vi "Mode Page.vi"(8 "Error in":errorcluster, 11 "INL DNL Test in":refnum<class "INL DNL Test.lvclass">) -> (0 "Error out":errorcluster, 3 "INL DNL Test out":refnum<class "INL DNL Test.lvclass">)   [LabVIEW 2020, in "INL DNL Test.lvclass"]
uses:
  INL DNL Test.lvclass
  D:/SDLC/Class/INL DNL Test/Test/Parent/Test.lvclass
  Typedef/User event controls.ctl
  Device/Parent/Device.lvclass
  DNL INL Test.lvlib
panel:
  out "number (0 to 1)":dbl
  in  "Error Rate":dbl
  in  "Voltage":dbl
  in  "Resolution":dbl
  in  "Digital to Analog converter":bool
  in  "Analog to digital converter":bool
  # "Choose the mode"
  # "Enter parameters"
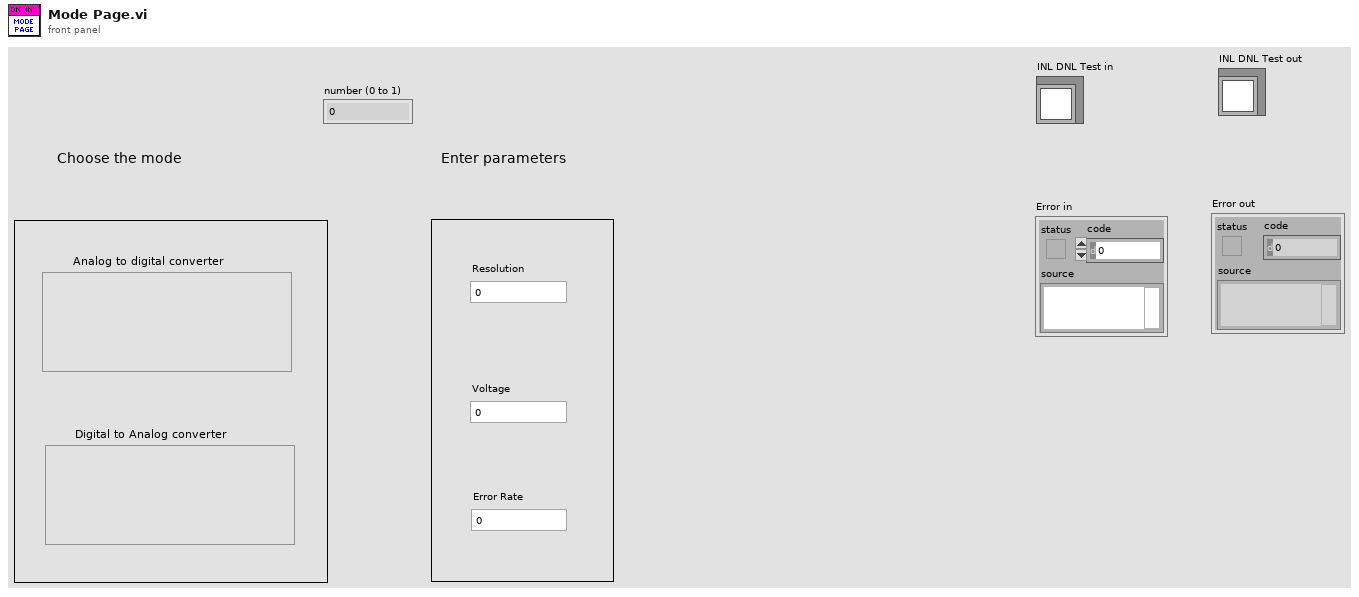
[diagram p1: front panel]
types:
  T1 = typedef "DNL INL Test.lvlib/User event controls.ctl" = enum16{"Create", "Generate", "Get Ref", "Destroy"}
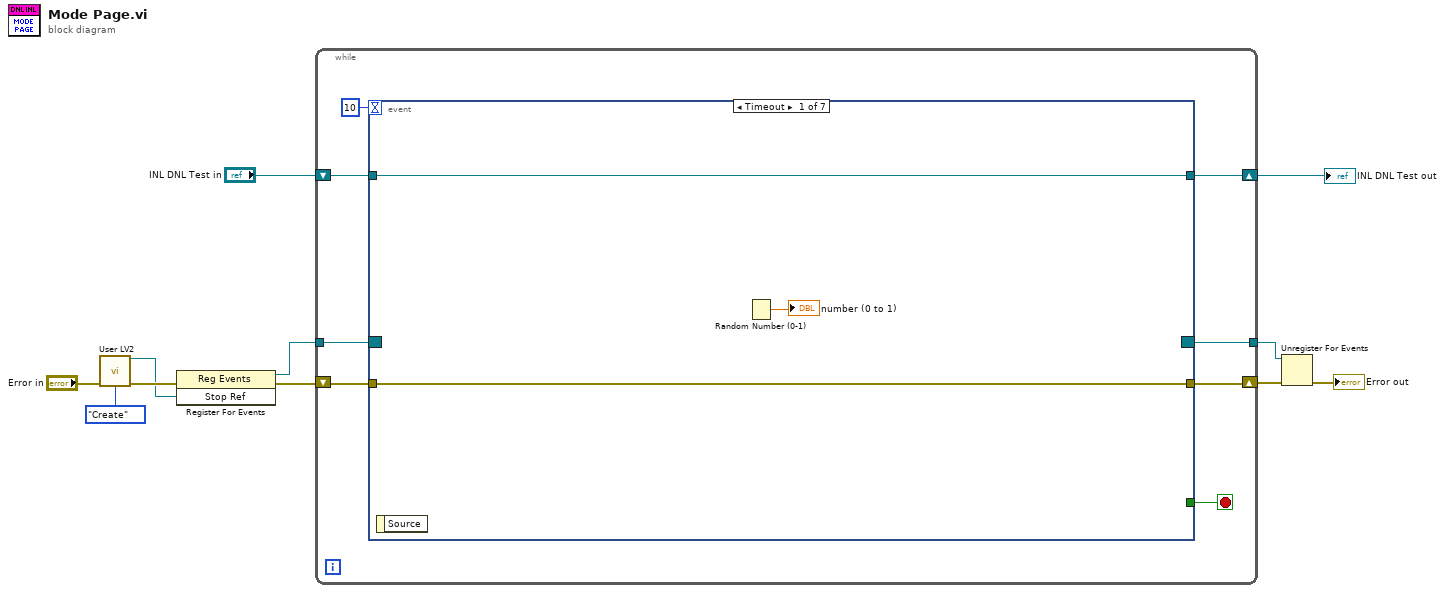
[diagram p0: block diagram]
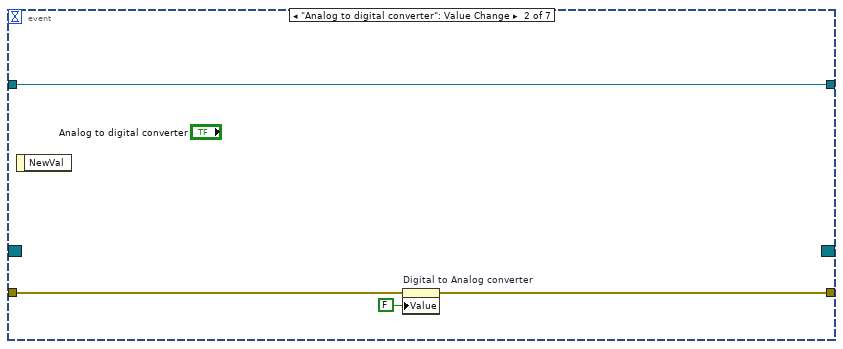
[diagram p2: hidden frame]
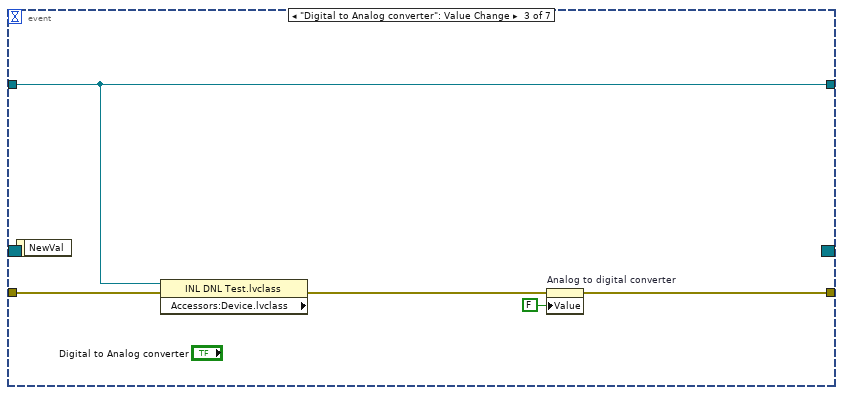
[diagram p3: hidden frame]
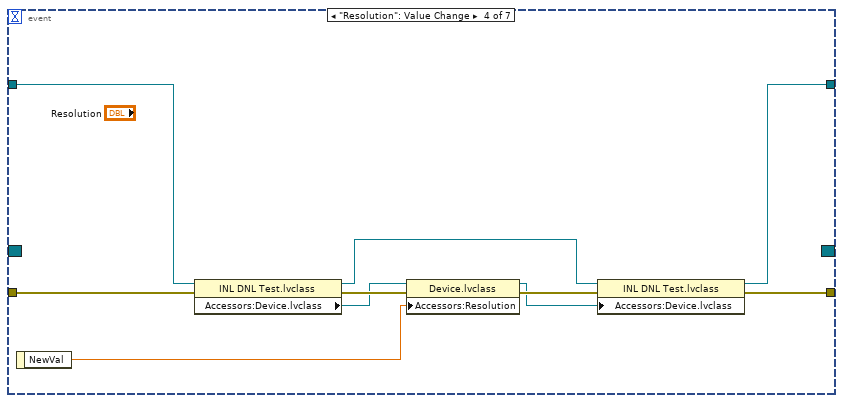
[diagram p4: hidden frame]
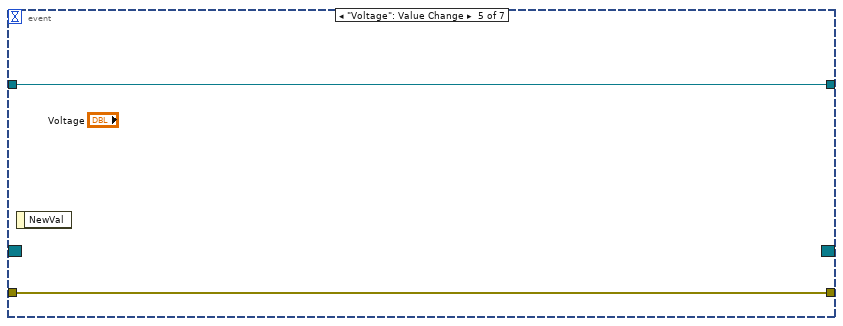
[diagram p5: hidden frame]
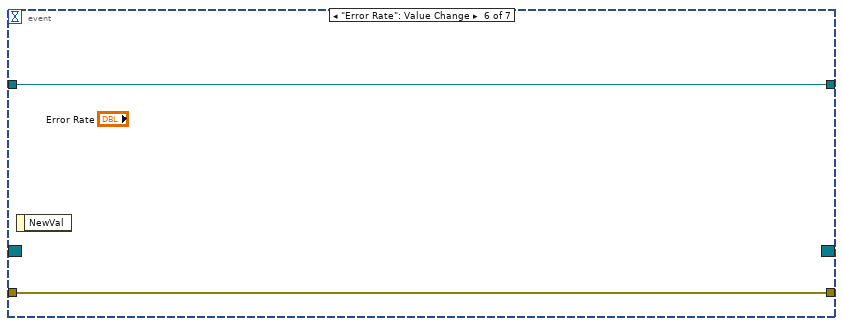
[diagram p6: hidden frame]
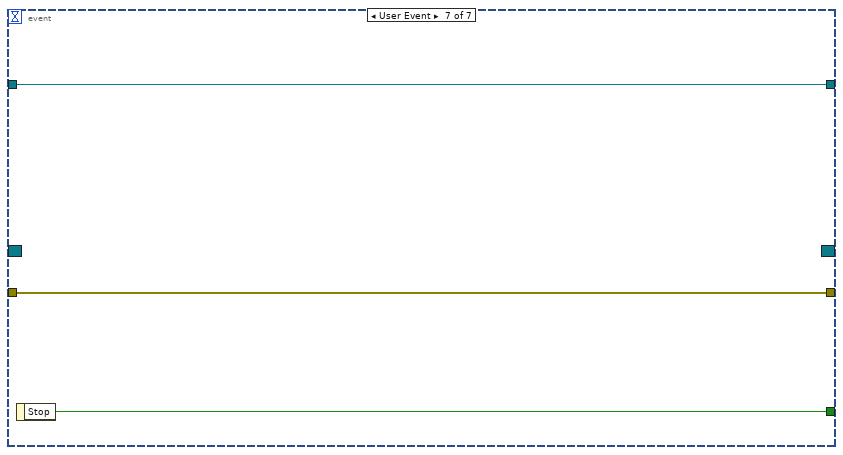
[diagram p7: hidden frame]
diagram:
  n1 = call "User LV2.vi"("Error In"="Error in", "User event controls"=User_event_controls."Create") -> ("Stop Ref"=w8:refnum<user-event>, "Error Out"=w9:errorcluster)  [unwired: 12 in]
  n2 = register-events(error in=w9, w8) -> (reference out=w7:refnum<event-registration>, error out=w6:errorcluster)  [unwired: 1 in]
  n3 = while {
    tunnel: w7 -> [w18]
    shift-right: [w15] -> w4
    shift-left: "INL DNL Test in" -> [w16]
    shift-right: [w13] -> w3
    shift-left: w6 -> [w17]
    tunnel: [w12] -> w1
    stop <- w14 stop-if-true
    n4 = event shown="[0] Timeout" {
      selector: w18 -> [_ _ _ _ _ _ _]
      dyn-events: [_ _ _ _ _ _ _] -> w12
      timeout: 10 -> [_ _ _ _ _ _ _]
      tunnel: w17 -> [w21 w25 w31 w41 w42 w44 w46]
      tunnel: w16 -> [w22 w26 w29 w39 w43 w45 w48]
      tunnel: [w22 w26 w29 w32 w43 w45 w48] -> w15
      tunnel: [_ _ _ _ _ _ w47] -> w14
      tunnel: [w21 w24 w28 w35 w42 w44 w46] -> w13
      event Timeout {
        n5 = event-data() -> ()  [unwired: 1 in, 1 out]
        n6 = Random Number (0-1)() -> (number: 0 to 1=→"number (0 to 1)":dbl)
      }
      event "Analog to digital converter": Value Change {
        n7 = event-data() -> ()  [unwired: 1 in, 1 out]
        n8 = property on="Digital to Analog converter" class="Bool (strict)"(error in=w25, "Value"=FALSE ("Digital to Analog converter")) -> (error out=w24:errorcluster)  [unwired: 1 in, 1 out]
      }
      event "Digital to Analog converter": Value Change {
        n9 = event-data() -> ()  [unwired: 1 in, 1 out]
        n10 = property class="INL DNL Test.lvclass" props=["Accessors:Device.lvclass"](reference=w29, error in=w31) -> (error out=w30:errorcluster)  [unwired: 2 out]
        n11 = property on="Analog to digital converter" class="Bool (strict)"(error in=w30, "Value"=FALSE ("Analog to digital converter")) -> (error out=w28:errorcluster)  [unwired: 1 in, 1 out]
      }
      event "Resolution": Value Change {
        n12 = event-data() -> ("NewVal"=w36:dbl)  [unwired: 1 in]
        n13 = property class="INL DNL Test.lvclass"(reference=w39, error in=w41) -> (reference out=w34:refnum<class "INL DNL Test.lvclass">, error out=w40:errorcluster, "Accessors:Device.lvclass"=w37:refnum<class "Device.lvclass">)
        n14 = property class="Device.lvclass"(reference=w37, error in=w40, "Accessors:Resolution"=w36) -> (reference out=w33:refnum<class "Device.lvclass">, error out=w38:errorcluster)
        n15 = property class="INL DNL Test.lvclass"(reference=w34, error in=w38, "Accessors:Device.lvclass"=w33) -> (reference out=w32:refnum<class "INL DNL Test.lvclass">, error out=w35:errorcluster)
      }
      event "Voltage": Value Change {
        n16 = event-data() -> ()  [unwired: 1 in, 1 out]
      }
      event "Error Rate": Value Change {
        n17 = event-data() -> ()  [unwired: 1 in, 1 out]
      }
      event User Event {
        n18 = event-data() -> ("Stop"=w47:bool)  [unwired: 1 in]
      }
    }
  }
  "INL DNL Test out" <- w4
  n19 = Unregister For Events(event registration refnum=w1, error in=w3) -> (error out=→"Error out":errorcluster)
